vi "Write Next State.vi"(8 "error in (no error)":errorcluster, 10 "New_State":string, 11 "State Machine in":refnum<class "State Machine.lvclass">) -> (0 "error out":errorcluster, 3 "State Machine out":refnum<class "State Machine.lvclass">)   [LabVIEW 2018, in "State Machine.lvclass"]
uses:
  State Machine.lvclass
  State Machine.lvclass/State Machine.ctl
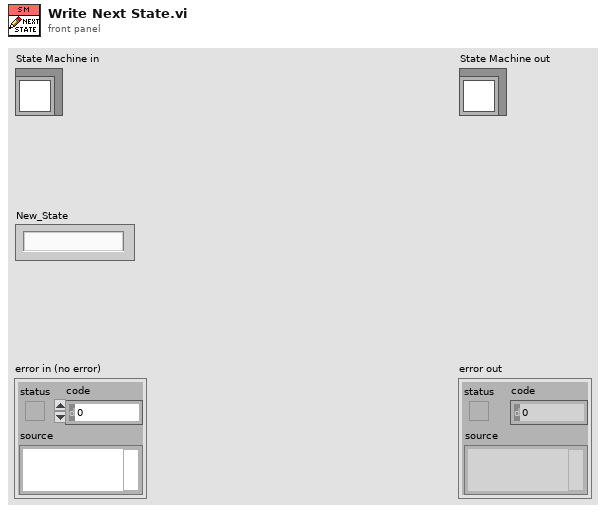
[diagram p1: front panel]
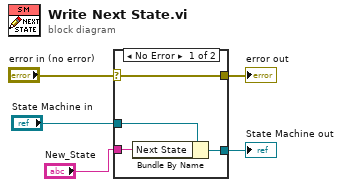
[diagram p0: block diagram]
diagram:
  n1 = case shown="No Error" "error in (no error)" {
    selector: "error in (no error)" -> [w6 w11]
    tunnel: [w6 w11] -> w2
    tunnel: [w7 w10] -> w3
    tunnel: "State Machine in" -> [w9 w10]
    tunnel: "New_State" -> [w8 _]
    frame No Error {
      n2 = Bundle By Name(cluster=w9, "Next State"=w8) -> (w7:refnum<class "State Machine.lvclass">)
    }
    frame Error {
    }
  }
  "error out" <- w2
  "State Machine out" <- w3
